vi "单步测试一键复位.vi"(8 "Error in":errorcluster) -> (0 "error out":errorcluster)   [LabVIEW 2016, in "斯坦道CODMn.lvlib"]
uses:
  <vilib>/Plasmionique/MB Master/MB Master.lvlib
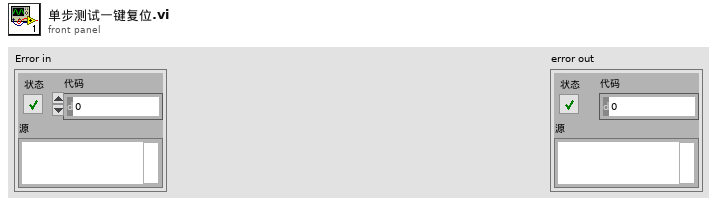
[diagram p1: front panel]
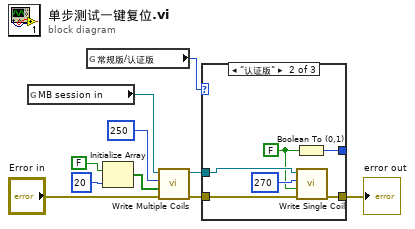
[diagram p0: block diagram]
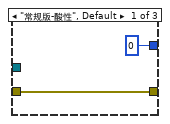
[diagram p2: hidden frame]
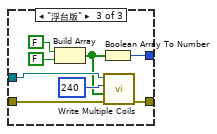
[diagram p3: hidden frame]
diagram:
  n1 = global read "COD浓度全局变量.vi" "MB session in"() -> (w7:refnum<class "MB_Master.lvclass">)
  n2 = global read "CODMn断电保存全局变量.vi" "常规版/认证版"() -> (w2:enum16{"常规版-酸性", "常规版-碱性", "认证版", "浮台版"})
  n3 = Initialize Array(FALSE, 20 ("维数大小")) -> (w5:bool[])
  n4 = call <vilib>:"Write Multiple Coils.vi"("error in (no error)"="Error in", "values"=w5, "starting address"=u16 250, "MB session in"=w7) -> ("error out"=w3:errorcluster, "MB session out"=w4:refnum<class "MB_Master.lvclass">)  [unwired: 6 in]
  n5 = case shown="\"认证版\"" w2 {
    tunnel: w4 -> [_ w18 w26]
    tunnel: w3 -> [w12 w17 w25]
    tunnel: [w12 w15 w21] -> w1
    tunnel: [u32 0 w13 w19] -> _
    frame "常规版-酸性", Default {
    }
    frame "认证版" {
      w14 = FALSE ("高锰酸钾滴定（10uL每滴）")
      n6 = Boolean To (0,1)(Boolean=w14) -> (0, 1=w13:i16)
      n7 = call <vilib>:"Write Single Coil.vi"("error in (no error)"=w17, "value"=w14, "address"=u16 270 ("starting address"), "MB session in"=w18) -> ("error out"=w15:errorcluster)  [unwired: 6 in, 1 out]
    }
    frame "浮台版" {
      n8 = Build Array(FALSE ("采水泵进"), FALSE ("采水泵排")) -> (w20:bool[])
      n9 = Boolean Array To Number(Boolean array=w20) -> (number=w19:u32)
      n10 = call <vilib>:"Write Multiple Coils.vi"("error in (no error)"=w25, "values"=w20, "starting address"=u16 240, "MB session in"=w26) -> ("error out"=w21:errorcluster)  [unwired: 6 in, 1 out]
    }
  }
  "error out" <- w1
